vi "PPR_TRAJECTORY_EXECUTE_REL.vi"(8 "Init":bool, 9 "Max Wheel Speed M/S":dbl=2.5, 11 "Gyro Heading\nRAD":dbl) -> (0 "AtReference":bool, 1 "Position Error Ft":dbl, 2 "Right Speed Dmd M/S":dbl, 3 "Left Speed Dmd M/S":dbl)   [LabVIEW 2019]
uses:
  <vilib>/Rock Robotics/WPI/ThirdParty/MJansen/PathPlanner/TypeDef/PathPlannerTrajectory.ctl
  <vilib>/Rock Robotics/WPI/ThirdParty/MJansen/PathPlanner/TypeDef/PathPlannerTrajectoryState.ctl
  <vilib>/Rock Robotics/WPI/ThirdParty/JAS_Junk/TrajLib/TypeDef/TRANSLATION2D.ctl
  <vilib>/Rock Robotics/WPI/ThirdParty/JAS_Junk/TrajLib/TypeDef/ROTATION2D.ctl
  <vilib>/Rock Robotics/WPI/ThirdParty/MJansen/PathPlanner/TypeDef/PathPlannerPathConstraints.ctl
  <vilib>/Rock Robotics/WPI/ThirdParty/JAS_Junk/TrajLib/VI/Util_GetTime_U32.vi
  <vilib>/Rock Robotics/WPI/ThirdParty/JAS_Junk/TrajLib/VI/DiffDrvOdom2_New.vi
  <vilib>/Rock Robotics/WPI/ThirdParty/JAS_Junk/TrajLib/VI/DiffDrvOdom2_Reset.vi
  <vilib>/Rock Robotics/WPI/ThirdParty/JAS_Junk/TrajLib/VI/DiffDrvOdom2_Update.vi
  <vilib>/Rock Robotics/WPI/ThirdParty/JAS_Junk/TrajLib/Rotation2d_GetRadians.vi
  <vilib>/Rock Robotics/SystemInterfaces/NetworkCommunication/NetComm_UsageReport_report.vi
  <vilib>/Rock Robotics/WPI/ThirdParty/JAS_Junk/TrajLib/Pose2d_getRotation.vi
  <vilib>/Rock Robotics/WPI/ThirdParty/JAS_Junk/TrajLib/Rotation2d_Minus.vi
  <vilib>/Rock Robotics/WPI/ThirdParty/JAS_Junk/TrajLib/Rotation2d_Plus.vi
  <vilib>/Rock Robotics/WPI/ThirdParty/JAS_Junk/TrajLib/Twist2d_Create.vi
  <vilib>/Rock Robotics/WPI/ThirdParty/JAS_Junk/TrajLib/Rotation2d_UnaryMinus.vi
  <vilib>/Rock Robotics/WPI/ThirdParty/JAS_Junk/TrajLib/Rotation2d_RotateBy.vi
  <vilib>/Rock Robotics/WPI/ThirdParty/JAS_Junk/TrajLib/Rotation2d_CreateXY.vi
  <vilib>/Rock Robotics/WPI/ThirdParty/JAS_Junk/TrajLib/Util_CalcDist.vi
  <vilib>/Rock Robotics/WPI/ThirdParty/JAS_Junk/TrajLib/VI/Util_GetTime_U64.vi
  PPR_TRAJECTORY_GLOBALS.vi
  Diff_Drive_System/PPR_DRIVE_GLOBALS.vi
  <vilib>/Rock Robotics/WPI/ThirdParty/JAS_Junk/TrajLib/Globals/Util_LibraryGlobals.vi
  <vilib>/Rock Robotics/WPI/ThirdParty/JAS_Junk/TrajLib/Pose2d_Exp.vi
  <vilib>/Rock Robotics/WPI/ThirdParty/JAS_Junk/TrajLib/Trajectory_Library.lvlib
  <vilib>/Rock Robotics/WPI/ThirdParty/MJansen/PathPlanner/PathPlanner24.lvlib
panel:
  out "PathPlannerTrajectory":T1 {"States"."TargetHolonomicRotation"."SIN" format="%13.4f"; "States"."TargetHolonomicRotation"."COS" format="%13.4f"; "States"."TargetHolonomicRotation"."VALUE" format="%13.4f"; "States"."Heading"."SIN" format="%13.4f"; "States"."Heading"."COS" format="%13.4f"; "States"."Heading"."VALUE" format="%13.4f"; "States"."PositionMeters"."Y" format="%14.3f"; "States"."PositionMeters"."X" format="%14.3f"}
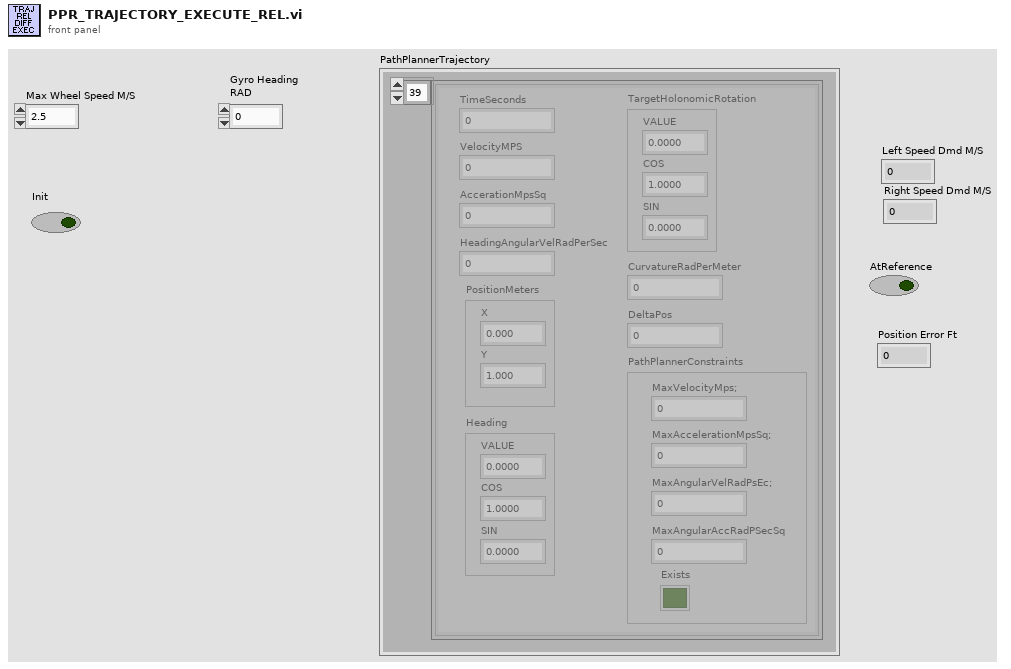
[diagram p1: front panel]
types:
  T1 = typedef "PathPlanner24.lvlib/PathPlannerTrajectory.ctl" = cluster{"States":T2[]}
  T2 = typedef "PathPlanner24.lvlib/PathPlannerTrajectoryState.ctl" = cluster{"TimeSeconds":dbl, "VelocityMPS":dbl, "AccerationMpsSq":dbl, "HeadingAngularVelRadPerSec":dbl, "PositionMeters":T3, "Heading":T4, "TargetHolonomicRotation":T4, "CurvatureRadPerMeter":dbl, "PathPlannerConstraints":T5, "DeltaPos":dbl}
  T3 = typedef "Trajectory_Library.lvlib/TRANSLATION2D.ctl" = cluster{"X":dbl, "Y":dbl}
  T4 = typedef "Trajectory_Library.lvlib/ROTATION2D.ctl" = cluster{"VALUE":dbl, "COS":dbl, "SIN":dbl}
  T5 = typedef "PathPlanner24.lvlib/PathPlannerPathConstraints.ctl" = cluster{"MaxVelocityMps;":dbl, "MaxAccelerationMpsSq;":dbl, "MaxAngularVelRadPsEc;":dbl, "MaxAngularAccRadPSecSq":dbl, "Exists":bool}
  T6 = typedef "Trajectory_Library.lvlib/POSE2D.ctl" = cluster{"TRANSLATION":T3, "ROTATION":T4}
  T7 = typedef "Trajectory_Library.lvlib/DIFF_DRIVE_KINEMATICS.ctl" = cluster{"TrackWidth_Meters":dbl}
  T8 = typedef "Trajectory_Library.lvlib/RAMSETE_EXE_TUNING.ctl" = cluster{"B":dbl, "Zeta":dbl, "X Tolerance M":dbl, "Y Tolerance M":dbl, "Heading Tolerance RAD":dbl, "Track Width M":dbl, "Max Speed M/S":dbl}
  T9 = typedef "Trajectory_Library.lvlib/RAMSETE.ctl" = cluster{"B":dbl, "Zeta":dbl, "poseTolerance":T6, "poseError":T6, "Enabled":bool}
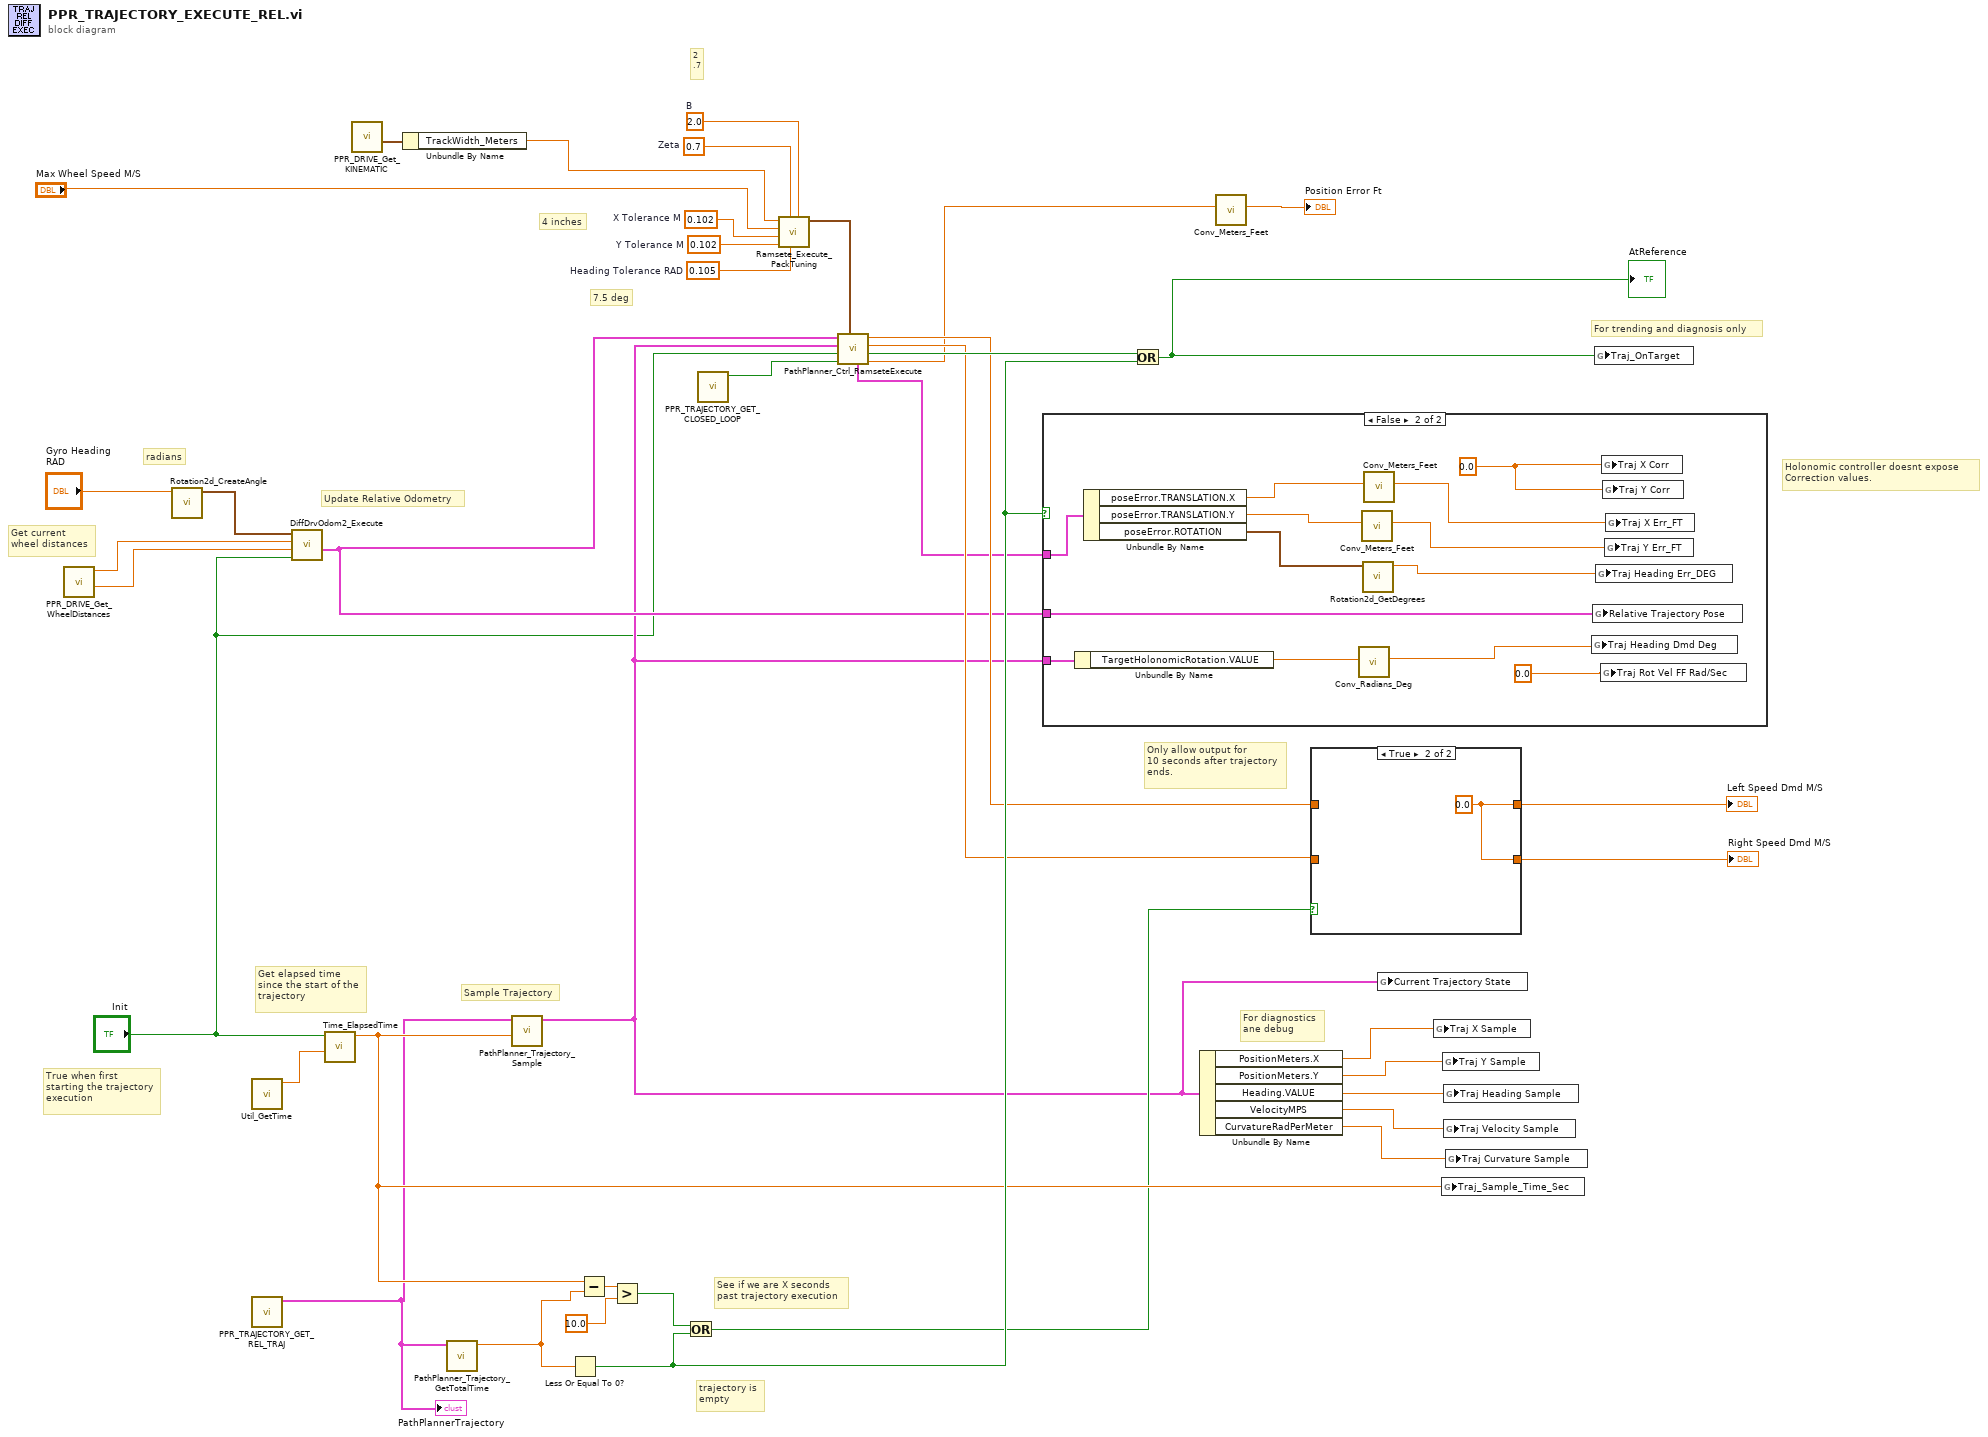
[diagram p0: block diagram]
diagram:
  w20 = 0.102  # X Tolerance M
  w21 = 0.102  # Y Tolerance M
  w22 = 0.7  # Zeta
  w23 = 0.105  # Heading Tolerance RAD
  w24 = 2.0  # B
  # "4 inches"
  # "7.5 deg"
  # "2\n.7"
  # "Get current \nwheel distances"
  # "Update Relative Odometry"
  # "radians"
  # "trajectory is \nempty"
  # "True when first\nstarting the trajectory\nexecution"
  # "Get elapsed time\nsince the start of the\ntrajectory"
  # "Holonomic controller doesnt expose\nCorrection values."
  # "For trending and diagnosis only"
  # "For diagnostics\nane debug"
  # "Sample Trajectory"
  # "See if we are X seconds \npast trajectory execution"
  # "Only allow output for\n10 seconds after trajectory\nends."
  n1 = call "PPR_DRIVE_Get_WheelDistances.vi"() -> ("Right Wheel Dist M"=w14:dbl, "Left Wheel Dist M"=w15:dbl)  [unwired: 10 in]
  n2 = call <vilib>:"Rotation2d_CreateAngle.vi"("Angle"="Gyro Heading\nRAD") -> ("ROTATION"=w16:T4)  [unwired: 10 in]
  n3 = call <vilib>:"Util_GetTime.vi"() -> ("FPGA_Time_Seconds"=w38:dbl)  [unwired: 9 in, 2 out]
  n4 = call "PPR_TRAJECTORY_GET_REL_TRAJ.vi"() -> ("Relative_Trajectory"=w27:T1)  [unwired: 11 in]
  "PathPlannerTrajectory" <- w27
  n5 = call <vilib>:"DiffDrvOdom2_Execute.vi"("Init / Reset"="Init", "Right Distance M"=w14, "Left Distance M"=w15, "Gyro Reading"=w16) -> ("Pose Meters"=w5:T6)  [unwired: 6 in, 1 out]
  n6 = call <vilib>:"Time_ElapsedTime.vi"("PassthroughTime_SEC"=w38, "Reset"="Init") -> ("Elapsed Time Sec"=w29:dbl)  [unwired: 9 in]
  n7 = call "PPR_DRIVE_Get_KINEMATIC.vi"() -> ("out DIFF_DRIVE_KINEMATICS"=w19:T7)  [unwired: 11 in]
  n8 = Unbundle By Name(w19) -> ("TrackWidth_Meters"=w18:dbl)
  n9 = call <vilib>:"PathPlanner_Trajectory_GetTotalTime.vi"("PathPlannerTrajectory"=w27) -> ("TotalTimeSeconds"=w28:dbl)  [unwired: 10 in]
  n10 = call <vilib>:"PathPlanner_Trajectory_Sample.vi"("Time"=w29, "PathPlannerTrajectory"=w27) -> ("PathPlannerState"=w4:T2)  [unwired: 9 in]
  n11 = Less Or Equal To 0?(x=w28) -> (x <= 0?=w30:bool)
  n12 = Subtract(x=w29, y=w28) -> (x-y=w40:dbl)
  n13 = Greater?(x=w40, y=10.0) -> (0:w32:bool)
  n14 = Or(x=w32, y=w30) -> (x .or. y?=w11:bool)
  n15 = call "PPR_TRAJECTORY_GET_CLOSED_LOOP.vi"() -> ("AUTO_CLOSED_LOOP"=w2:bool)  [unwired: 11 in]
  n16 = call <vilib>:"Ramsete_Execute_PackTuning.vi"("B"=w24, "Heading Tolerance RAD"=w23, "Zeta"=w22, "Y Tolerance M"=w21, "X Tolerance M"=w20, "Max Speed M/S"="Max Wheel Speed M/S", "Track Width M"=w18) -> ("RAMSETE_EXE_TUNING"=w25:T8)  [unwired: 4 in]
  n17 = call <vilib>:"PathPlanner_Ctrl_RamseteExecute.vi"("RAMSETE_EXE_TUNING SI"=w25, "Enabled"=w2, "Reset"="Init", "PathPlannerState"=w4, "Current Pose SI"=w5) -> ("Position Error M"=w7:dbl, "At Reference"=w17:bool, "Right Speed Dmd M/S"=w8:dbl, "Left Speed Dmd M/S"=w9:dbl, "outRAMSETE"=w1:T9)  [unwired: 2 in]
  n18 = case shown="False" w30 {
    tunnel: w5 -> [_ w43]
    tunnel: w1 -> [_ w49]
    tunnel: w4 -> [_ w46]
    frame True {
    }
    frame False {
      w53 = 0.0 ("Y Corr")
      n19 = Unbundle By Name(w46) -> ("TargetHolonomicRotation.VALUE"=w45:dbl)
      n20 = Unbundle By Name(w49) -> ("poseError.TRANSLATION.X"=w48:dbl, "poseError.TRANSLATION.Y"=w47:dbl, "poseError.ROTATION"=w41:T4)
      n21 = call <vilib>:"Conv_Radians_Deg.vi"("Radians"=w45) -> ("Degrees"=w44:dbl)  [unwired: 10 in]
      n22 = call <vilib>:"Conv_Meters_Feet.vi"("Meters"=w47) -> ("Feet"=w52:dbl)  [unwired: 10 in]
      n23 = call <vilib>:"Rotation2d_GetDegrees.vi"("in ROTATION"=w41) -> ("AngleDegrees"=w42:dbl)  [unwired: 10 in]
      n24 = call <vilib>:"Conv_Meters_Feet.vi"("Meters"=w48) -> ("Feet"=w51:dbl)  [unwired: 10 in]
      n25 = global write "PPR_TRAJECTORY_GLOBALS.vi" "Traj Heading Dmd Deg"(w44) -> ()
      n26 = global write "PPR_TRAJECTORY_GLOBALS.vi" "Relative Trajectory Pose"(w43) -> ()
      n27 = global write "PPR_TRAJECTORY_GLOBALS.vi" "Traj Heading Err_DEG"(w42) -> ()
      n28 = global write "PPR_TRAJECTORY_GLOBALS.vi" "Traj Rot Vel FF Rad/Sec"(0.0 ("Traj Heading Dmd Deg")) -> ()
      n29 = global write "PPR_TRAJECTORY_GLOBALS.vi" "Traj X Corr"(w53) -> ()
      n30 = global write "PPR_TRAJECTORY_GLOBALS.vi" "Traj Y Corr"(w53) -> ()
      n31 = global write "PPR_TRAJECTORY_GLOBALS.vi" "Traj Y Err_FT"(w52) -> ()
      n32 = global write "PPR_TRAJECTORY_GLOBALS.vi" "Traj X Err_FT"(w51) -> ()
    }
  }
  n33 = Or(x=w17, y=w30) -> (x .or. y?=w31:bool)
  "AtReference" <- w31
  n34 = Unbundle By Name(w4) -> ("PositionMeters.X"=w37:dbl, "PositionMeters.Y"=w36:dbl, "Heading.VALUE"=w35:dbl, "VelocityMPS"=w34:dbl, "CurvatureRadPerMeter"=w33:dbl)
  n35 = call <vilib>:"Conv_Meters_Feet.vi"("Meters"=w7) -> ("Feet"=→"Position Error Ft":dbl)  [unwired: 10 in]
  n36 = case shown="True" w11 {
    tunnel: w9 -> [w55 _]
    tunnel: [w55 w56] -> w13
    tunnel: w8 -> [w54 _]
    tunnel: [w54 w56] -> w12
    frame False {
    }
    frame True {
      w56 = 0.0 ("vX")
    }
  }
  "Left Speed Dmd M/S" <- w13
  "Right Speed Dmd M/S" <- w12
  n37 = global write "PPR_TRAJECTORY_GLOBALS.vi" "Current Trajectory State"(w4) -> ()
  n38 = global write "PPR_TRAJECTORY_GLOBALS.vi" "Traj X Sample"(w37) -> ()
  n39 = global write "PPR_TRAJECTORY_GLOBALS.vi" "Traj_Sample_Time_Sec"(w29) -> ()
  n40 = global write "PPR_TRAJECTORY_GLOBALS.vi" "Traj Y Sample"(w36) -> ()
  n41 = global write "PPR_TRAJECTORY_GLOBALS.vi" "Traj Heading Sample"(w35) -> ()
  n42 = global write "PPR_TRAJECTORY_GLOBALS.vi" "Traj Velocity Sample"(w34) -> ()
  n43 = global write "PPR_TRAJECTORY_GLOBALS.vi" "Traj Curvature Sample"(w33) -> ()
  n44 = global write "PPR_TRAJECTORY_GLOBALS.vi" "Traj_OnTarget"(w31) -> ()
